vi "ForceWait.vi"() -> ()   [LabVIEW 2011]
panel:
  in  "ForceWait":bool
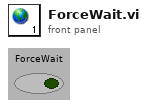
[diagram p1: front panel]
diagram:
